vi "Periodic Tasks.vi"(8 "error in":errorcluster) -> ()   [LabVIEW 2019]
doc: "This VI runs in parallel to other robot code. It can contain as many user-defined periodic loops as you need. These can carry out PID or other sorts of timed response."
uses:
  <vilib>/Rock Robotics/WPI/Utilities/WPI_GetSetVariantRefNum.vi
  Robot Global Data.vi
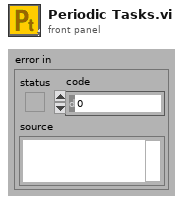
[diagram p1: front panel]
types:
  T1 = typedef "WPI_JoystickDevRef.ctl" = cluster{"Device":T2}
  T2 = typedef "WPI_JoystickDeviceEnum.ctl" = enum16{"USB 0", "USB 1", "USB 2", "USB 3", "USB 4", "USB 5"}
  T3 = cluster{"JoystickDevRef":T1, "JoystickDevRef":T1}
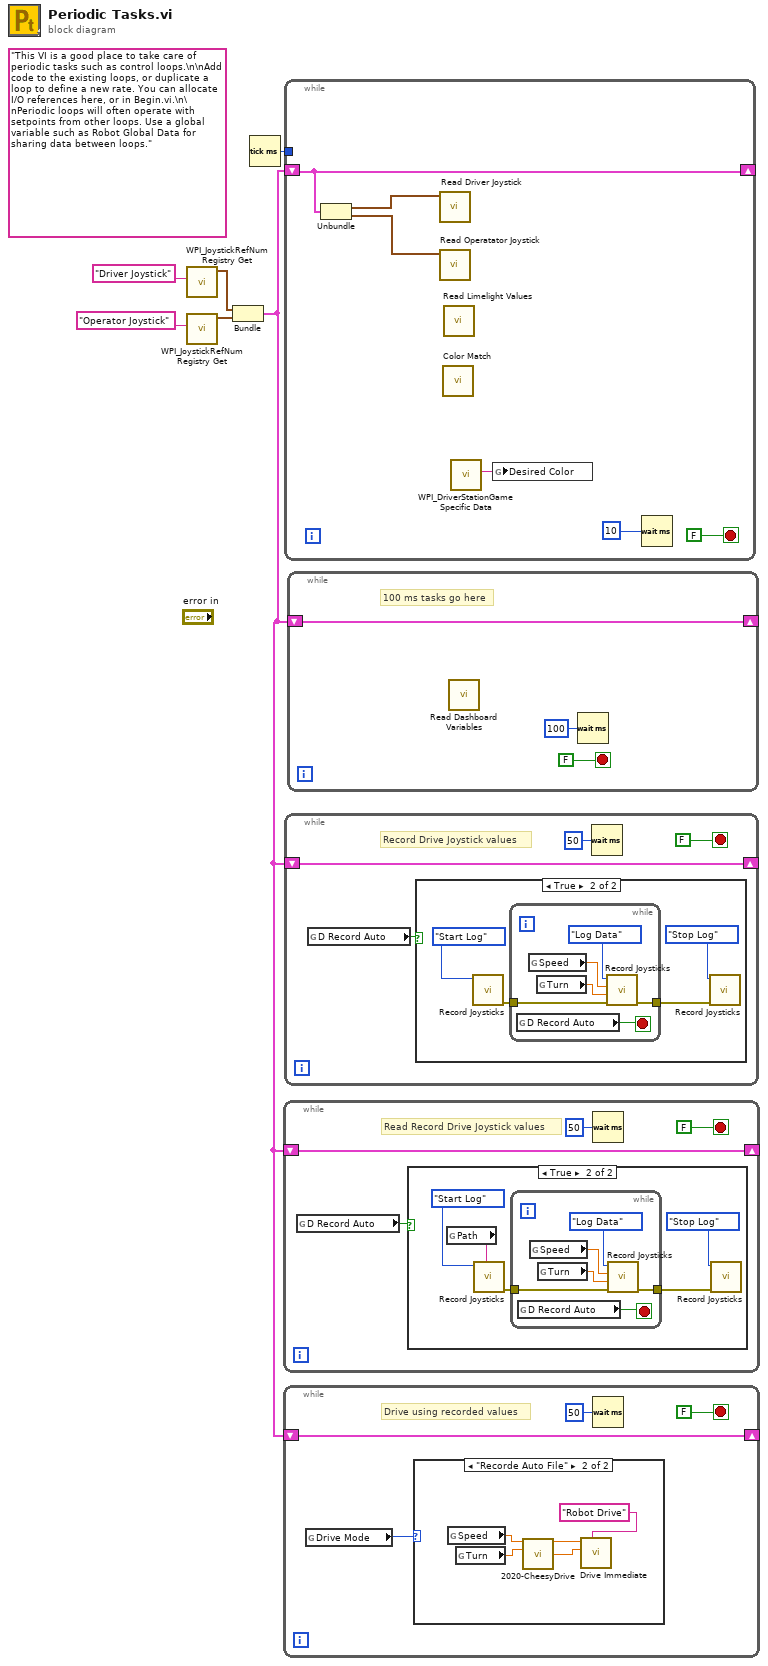
[diagram p0: block diagram]
diagram:
  (unwired) "This VI is a good place to take care of periodic tasks such as control loops.\n\nAdd code to the existing loops, or duplicate a loop to define a new rate. You can allocate I/O references here, or in Begin.vi.\n\nPeriodic loops will often operate with setpoints from other loops. Use a global variable such as Robot Global Data for sharing data between loops."
  n1 = call <vilib>:"WPI_JoystickRefNum Registry Get.vi"("refnum name"="Driver Joystick") -> ("JoystickDevRef"=w2:T1)  [unwired: 1 in, 9 out]
  n2 = call <vilib>:"WPI_JoystickRefNum Registry Get.vi"("refnum name"="Operator Joystick") -> ("JoystickDevRef"=w3:T1)  [unwired: 1 in, 9 out]
  n3 = Bundle("JoystickDevRef"=w2, "JoystickDevRef"=w3) -> (w1:T3)  [unwired: 1 in]
  n4 = Tick Count (ms)() -> (millisecond timer value=w5:u32)
  n5 = while {
    shift-right: [w8] -> _
    shift-left: w1 -> [w8]
    stop <- FALSE stop-if-true
    # "Read Record Drive Joystick values"
    n6 = global read "Robot Global Data.vi" "D Record Auto"() -> (w7:bool)
    n7 = case shown="True" w7 {
      frame False {
      }
      frame True {
        n8 = global read "Robot Global Data.vi" "Path"() -> (w11:string)
        n9 = call "Record Joysticks.vi"("Auto Name"=w11, "Function"=enum16{"Start Log", "Log Data", "Stop Log"}."Start Log") -> ("error out"=w15:errorcluster)  [unwired: 9 in]
        n10 = while {
          tunnel: w15 -> [w21]
          tunnel: [w20] -> w14
          stop <- w16 stop-if-true
          n11 = global read "Robot Global Data.vi" "D Record Auto"() -> (w16:bool)
          n12 = global read "Robot Global Data.vi" "Speed"() -> (w18:dbl)
          n13 = global read "Robot Global Data.vi" "Turn"() -> (w17:dbl)
          n14 = call "Record Joysticks.vi"("error in (no error)"=w21, "Turn X joystick"=w17, "Speed Y Joystick"=w18, "Function"=enum16{"Start Log", "Log Data", "Stop Log"}."Log Data") -> ("error out"=w20:errorcluster)  [unwired: 7 in]
        }
        n15 = call "Record Joysticks.vi"("error in (no error)"=w14, "Function"=enum16{"Start Log", "Log Data", "Stop Log"}."Stop Log") -> ()  [unwired: 9 in, 1 out]
      }
    }
    n16 = Wait (ms)(milliseconds to wait=u32 50) -> ()  [unwired: 1 out]
  }
  n17 = while {
    shift-right: [w23] -> _
    shift-left: w1 -> [w23]
    stop <- FALSE stop-if-true
    # "Drive using recorded values"
    n18 = global read "Robot Global Data.vi" "Drive Mode"() -> (w22:enum16{"Manual", "Recorde Auto File"})
    n19 = case shown="\"Recorde Auto File\"" w22 {
      frame "Manual", Default {
      }
      frame "Recorde Auto File" {
        n20 = global read "Robot Global Data.vi" "Speed"() -> (w30:dbl)
        n21 = global read "Robot Global Data.vi" "Turn"() -> (w29:dbl)
        n22 = call "2020-CheesyDrive.vi"("Throttle"=w30, "Wheel"=w29) -> ("Left PWM"=w28:dbl, "Right PWM"=w27:dbl)  [unwired: 12 in]
        n23 = call "Drive Immediate.vi"("Description"="Robot Drive", "Right Setpoint"=w27, "Left Setpoint"=w28) -> ()  [unwired: 8 in, 1 out]
      }
    }
    n24 = Wait (ms)(milliseconds to wait=u32 50) -> ()  [unwired: 1 out]
  }
  n25 = while {
    shift-right: [w34] -> _
    shift-left: w1 -> [w34]
    tunnel: w5 -> [_]
    stop <- FALSE stop-if-true
    n26 = Unbundle(w34) -> ("JoystickDevRef"=w33:T1, "JoystickDevRef"=w32:T1)
    n27 = call "Read Driver Joystick.vi"("Driver Joystick"=w33) -> ()  [unwired: 11 in]
    n28 = call "Read Operatator Joystick.vi"("Operator Joystick"=w32) -> ()  [unwired: 11 in]
    n29 = call "Color Match.vi"() -> ()  [unwired: 12 in]
    n30 = call "Read Limelight Values.vi"() -> ()  [unwired: 12 in]
    n31 = call <vilib>:"WPI_DriverStationGame Specific Data.vi"() -> ("Game Specific Data"=w31:string)  [unwired: 11 in]
    n32 = global write "Robot Global Data.vi" "Desired Color"(w31) -> ()
    n33 = Wait (ms)(milliseconds to wait=u32 10) -> ()  [unwired: 1 out]
  }
  n34 = while {
    shift-right: [w38] -> _
    shift-left: w1 -> [w38]
    stop <- FALSE stop-if-true
    # "Record Drive Joystick values"
    n35 = global read "Robot Global Data.vi" "D Record Auto"() -> (w37:bool)
    n36 = case shown="True" w37 {
      frame False {
      }
      frame True {
        n37 = call "Record Joysticks.vi"("Function"=enum16{"Start Log", "Log Data", "Stop Log"}."Start Log") -> ("error out"=w44:errorcluster)  [unwired: 10 in]
        n38 = while {
          tunnel: w44 -> [w50]
          tunnel: [w49] -> w43
          stop <- w45 stop-if-true
          n39 = global read "Robot Global Data.vi" "D Record Auto"() -> (w45:bool)
          n40 = global read "Robot Global Data.vi" "Speed"() -> (w47:dbl)
          n41 = global read "Robot Global Data.vi" "Turn"() -> (w46:dbl)
          n42 = call "Record Joysticks.vi"("error in (no error)"=w50, "Turn X joystick"=w46, "Speed Y Joystick"=w47, "Function"=enum16{"Start Log", "Log Data", "Stop Log"}."Log Data") -> ("error out"=w49:errorcluster)  [unwired: 7 in]
        }
        n43 = call "Record Joysticks.vi"("error in (no error)"=w43, "Function"=enum16{"Start Log", "Log Data", "Stop Log"}."Stop Log") -> ()  [unwired: 9 in, 1 out]
      }
    }
    n44 = Wait (ms)(milliseconds to wait=u32 50) -> ()  [unwired: 1 out]
  }
  n45 = while {
    shift-right: [w51] -> _
    shift-left: w1 -> [w51]
    stop <- FALSE stop-if-true
    # "100 ms tasks go here"
    n46 = call "Read Dashboard Variables.vi"() -> ()  [unwired: 12 in]
    n47 = Wait (ms)(milliseconds to wait=u32 100) -> ()  [unwired: 1 out]
  }
